vi "Send Hide GUI Message.vi"(8 "error in (no error)":errorcluster, 11 "Module in":refnum<class "Module.lvclass">) -> (0 "error out":errorcluster, 3 "Module out":refnum<class "Module.lvclass">)   [LabVIEW 2020, in "Volatus.lvlib" / "Module.lvclass"]
uses:
  Module.lvclass
  Module.lvclass/Module.ctl
  Volatus.lvlib
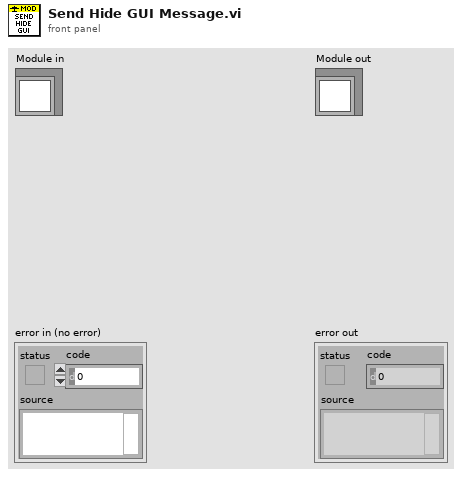
[diagram p1: front panel]
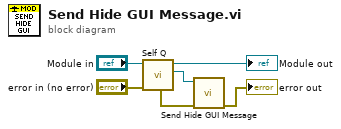
[diagram p0: block diagram]
diagram:
  n1 = call "Self Q.vi"("Module in"="Module in") -> ("Self Q"=w3:refnum<class "MessageQ.lvclass">, "Module out"=→"Module out":refnum<class "Module.lvclass">)  [unwired: 9 in]
  n2 = call "Send Hide GUI Message.vi"("error in (no error)"="error in (no error)", "MessageQ"=w3) -> ("error out"=→"error out":errorcluster)  [unwired: 9 in]
